vi "Get SS2 Data Bitness.vi"(10 "DAQ Parameters in":T1 {"# Gate Positions" format="%0.0f"; "Gate Offset" format="%0.0f"; "Bitness" format="%0.0f"; "# Gate Set" format="%0.0f"}, 11 "SS2 8-bit Frame Selection":T2 caption="SS2 Frame Selection") -> (2 "DAQ Parameters out":T1 {"# Gate Positions" format="%0.0f"; "Gate Offset" format="%0.0f"; "Bitness" format="%0.0f"; "# Gate Set" format="%0.0f"})   [LabVIEW 2021, in "SwissSPAD.lvlib"]
uses:
  SS2 DAQ Parameters.ctl
  SwissSPAD 8-bit Frames Read.ctl
  SwissSPAD.lvlib
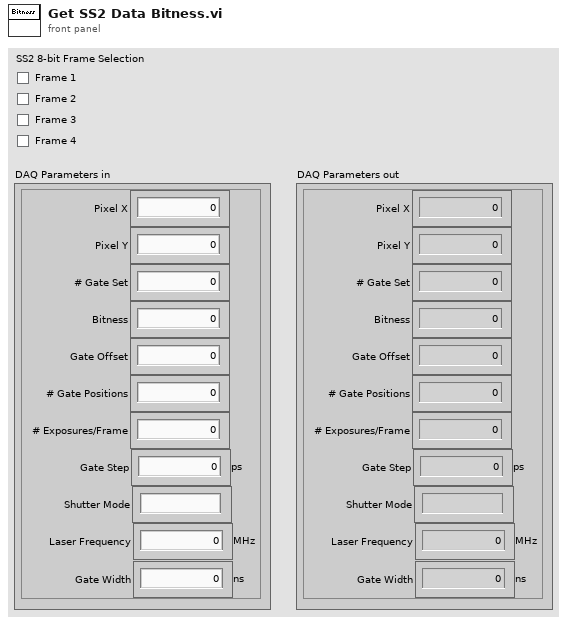
[diagram p1: front panel]
types:
  T1 = typedef "SwissSPAD.lvlib/SS2 DAQ Parameters.ctl" = cluster{"Pixel X":i32, "Pixel Y":i32, "# Gate Set":i32, "Bitness":i32, "Gate Offset":i32, "# Gate Positions":i32, "# Exposures/Frame ":i32, "Gate Step":dbl[unit], "Shutter Mode":string, "Laser Frequency":dbl[unit], "Gate Width":dbl[unit]}
  T2 = typedef "SwissSPAD.lvlib/SwissSPAD 8-bit Frames Read.ctl" = cluster{"Frame 1":bool, "Frame 2":bool, "Frame 3":bool, "Frame 4":bool}
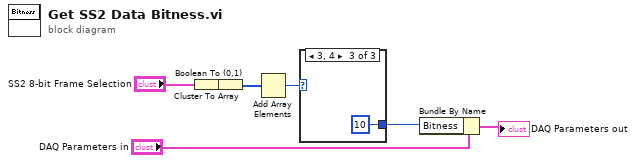
[diagram p0: block diagram]
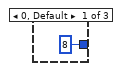
[diagram p2: hidden frame]
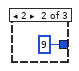
[diagram p3: hidden frame]
diagram:
  n1 = Cluster To Array(cluster="SS2 8-bit Frame Selection") -> (array=w6:bool[])
  n2 = Boolean To (0,1)(Boolean=w6) -> (0, 1=w5:i16[])
  n3 = Add Array Elements(numeric array=w5) -> (sum=w4:i16)
  n4 = case shown="3, 4" w4 {
    tunnel: [8 ("Bitness") 9 ("Bitness") 10 ("Bitness")] -> w1
    frame 0, Default {
    }
    frame 2 {
    }
    frame 3, 4 {
    }
  }
  n5 = Bundle By Name(cluster="DAQ Parameters in", "Bitness"=w1) -> (→"DAQ Parameters out":T1)
